vi "initialize Session Data.vi"(0 "OBJ - Session in":refnum<class "CVT.lvclass">, 11 "error in":errorcluster) -> (4 "OBJ - Session out":refnum<class "CVT.lvclass">, 15 "error out":errorcluster)   [LabVIEW 2016, in "CVT.lvclass"]
doc: "OVERRIDE VI\nPlaceholder for decendant sessions to initialize and set their default values"
uses:
  CVT.lvclass
  CVT.lvclass/CVT.ctl
  Write CVT.vi
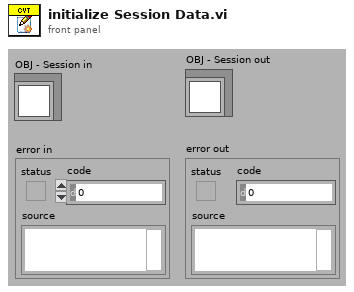
[diagram p1: front panel]
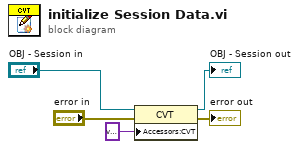
[diagram p0: block diagram]
diagram:
  n1 = property class="CVT"(reference="OBJ - Session in", error in="error in", "Accessors:CVT"=variant ("CVT")) -> (reference out=→"OBJ - Session out":refnum<class "CVT.lvclass">, error out=→"error out":errorcluster)
